vi "Query Gate delay.vi"(8 "error in (no error)":errorcluster, 10 "Gate (def: A)":T1, 11 "VISA resource name":refnum<visa-resource-name>) -> (0 "error out":errorcluster, 2 "output":dbl, 3 "VISA resource name out":refnum<visa-resource-name>)   [LabVIEW 2011, in "SR400.lvlib"]
doc: "GD i { ,t }\nThe GD command sets and reads the gate delays.\ni=0 or 1 designates A gate or B gate and is\nrequired. If t is included, the selected gate delay is\nset to t seconds where 0 <= t <= 999.2E-3. The\nresolution is variable depending upon the 4 most\nsignificant digits of t.\n4 most significant digits resolution in 4th digit\n1000 to 2048 1 (1001,1002,1003,...)\n2048 to 4096 2\n4096 to 8192 4\n8192 to 9992 8 (8192,8200,8208,...)\nFor example, near 10.00 ìs, the allowed values of\nt are 9.984 ìs, 9.992 ìs, 10.00 ìs, 10.01 ìs, etc.\nBelow 1.000 ìs, the resolution is 1 ns. Almost any\nvalue of t may be sent and the SR400 will round to\nthe nearest allowed value. If t is absent, the\nselected gate delay is returned. The gate delay may\nbe set and read regardless of the gate mode. If the\nmode is CW, the gate remains continuous. If the\nmode is SCAN, the GD command sets and reads\nthe starting position of the gate delay. Changing\nthe delay during a scan will cause the delay to be\nset to the new value on the next count period. Note\nthat the scan is not reset. Reading the delay during\na scan always returns the starting delay, not the\ncurrent delay."
uses:
  SR400.lvlib
  Typedefs/Gate.ctl
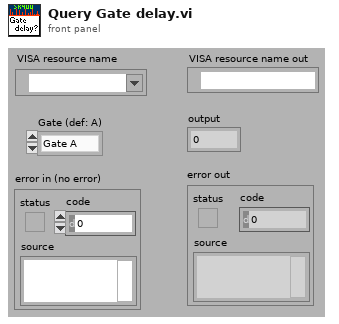
[diagram p1: front panel]
types:
  T1 = typedef "SR400.lvlib/Gate.ctl" = enum16{"Gate A", "Gate B"}
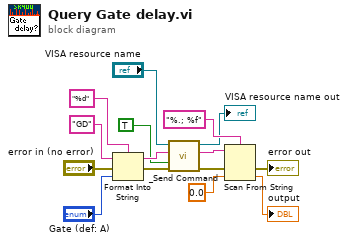
[diagram p0: block diagram]
diagram:
  n1 = Format Into String(format string="%d", initial string="GD" ("command"), error in="error in (no error)", "Gate (def: A)") -> (resulting string=w6:string, error out=w5:errorcluster)
  n2 = call "_Send Command.vi"("error in (no error)"=w5, "Query? (F)"=TRUE, "Command"=w6, "VISA resource name"="VISA resource name") -> ("error out"=w2:errorcluster, "Response"=w3:string, "VISA resource name out"=→"VISA resource name out":refnum<visa-resource-name>)  [unwired: 5 out]
  n3 = Scan From String(format string="%.; %f", input string=w3, error in=w2, default 1=0.0 ("default value 1")) -> (error out=→"error out":errorcluster, output 1=→"output":dbl)  [unwired: 1 in, 2 out]
